vi "Read Target XML-Files.vi"(5 "password":string, 7 "user name":string, 8 "error in (no error)":errorcluster, 9 "ddDestPath in":string, 10 "Target IP":string, 11 "protocol":T1=enum."WebDAV") -> (0 "error out":errorcluster, 2 "Fies":string[](array[string]), 3 "ddDestPath out":string)   [LabVIEW 2015, in "Scan Engine Custom Device.lvlib"]
uses:
  Scan Engine Custom Device.lvlib
  <resource>/Framework/Providers/indcomecat/_InternalSubVIs/_fileTransferProtocol.ctl
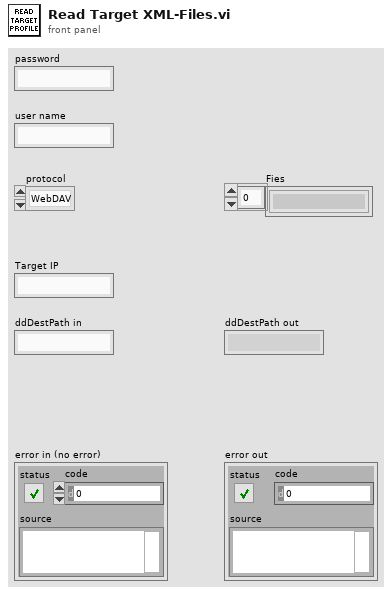
[diagram p1: front panel]
types:
  T1 = typedef "_fileTransferProtocol.ctl" = enum16{"Ftp", "WebDAV", "None"}
  T2 = typedef "_protocolSession.ctl" = cluster{"FTP session":T3, "WebDAV sssion":T4}
  T3 = typedef "NI_FTP.lvlib/FTP Session.ctl" = refnum<k5>
  T4 = typedef "NI_WebDAV.lvlib/SessionHandle.ctl" = refnum<k1>
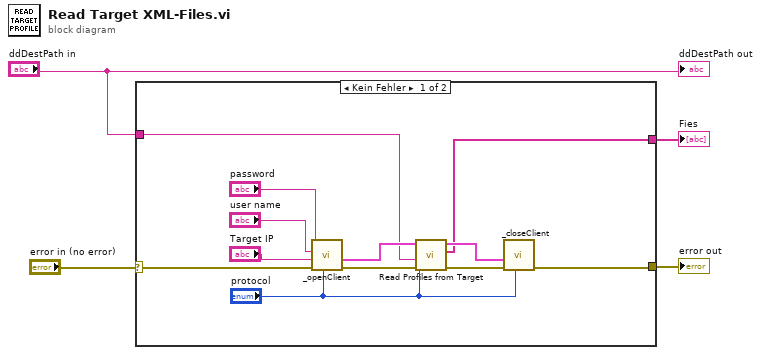
[diagram p0: block diagram]
diagram:
  n1 = case shown="Kein Fehler" "error in (no error)" {
    selector: "error in (no error)" -> [w15 w17]
    tunnel: [w16 w17] -> w3
    tunnel: "ddDestPath in" -> [w6 _]
    tunnel: [w5 _] -> w1
    frame No Error {
      n2 = call <resource>:"_openClient.vi"("protocol"="protocol", "error in (no error)"=w15, "Target IP"="Target IP", "user name"="user name", "password"="password") -> ("error out"=w14:errorcluster, "Cluster"=w7:T2)  [unwired: 5 in]
      n3 = call "Read Profiles from Target.vi"("error in (no error)"=w14, "directory path"=w6, "protocol"="protocol", "session in"=w7) -> ("error out"=w13:errorcluster, "Fies"=w5:string[], "session out"=w8:T2)  [unwired: 5 in]
      n4 = call <resource>:"_closeClient.vi"("protocol"="protocol", "error in"=w13, "session in"=w8) -> ("error out"=w16:errorcluster)  [unwired: 8 in]
    }
    frame Error {
    }
  }
  "error out" <- w3
  "Fies" <- w1
  "ddDestPath out" <- "ddDestPath in"
